vi "vsc_InstallPackage.vi"(8 "error in (no error)":errorcluster, 11 "CommandLine":path) -> (0 "error out":errorcluster, 2 "test details":string, 3 "output to action":string)   [LabVIEW 2017, in "_Try Beta Version of CSMF.lvlib"]
uses:
  _Try Beta Version of CSMF.lvlib
panel:
  out "output to action 2":string
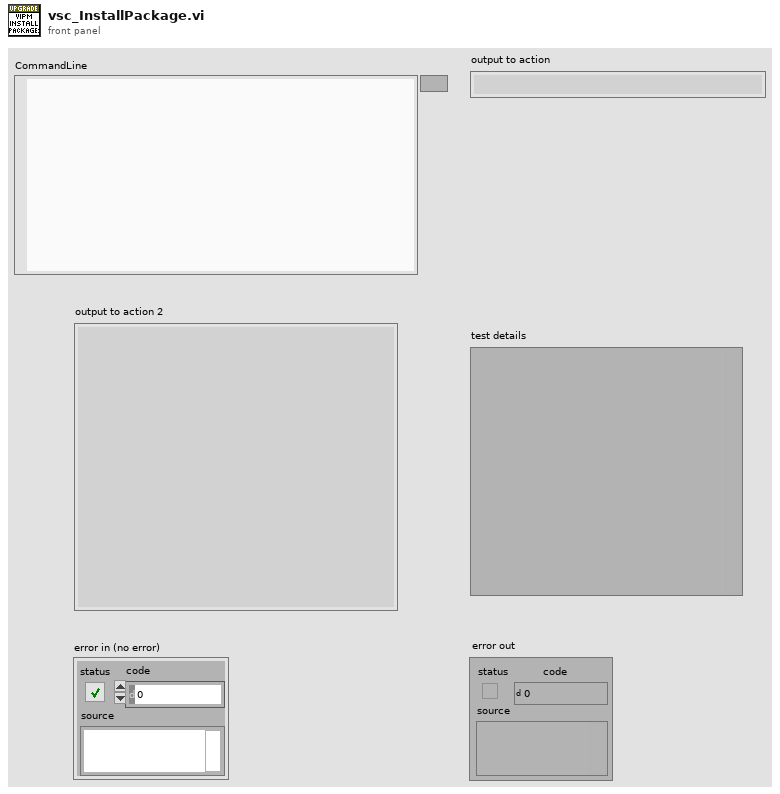
[diagram p1: front panel]
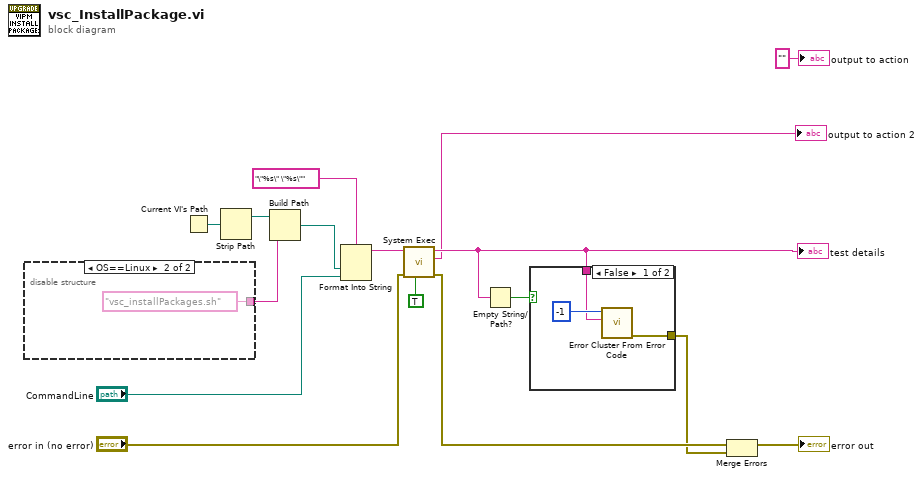
[diagram p0: block diagram]
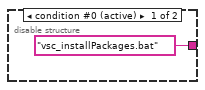
[diagram p2: hidden frame]
diagram:
  n1 = disable-structure shown="OS==Linux" {
    disable-tunnel: ["vsc_installPackages.bat" ("name or relative path") "vsc_installPackages.sh" ("name or relative path")] -> w8
    frame condition #0 (active) {
    }
    frame condition #1 {
    }
  }
  n2 = Current VI's Path() -> (path=w10:path)
  n3 = Strip Path(path=w10) -> (stripped path=w9:path)  [unwired: 1 out]
  n4 = Build Path(base path=w9, name or relative path=w8) -> (appended path=w7:path)
  n5 = Format Into String(format string="\"%s\" \"%s\"" ("command line"), w7, "CommandLine") -> (resulting string=w14:string)  [unwired: 2 in, 1 out]
  n6 = call <vilib>:"System Exec.vi"("run minimized? (F)"=TRUE, "error in (no error)"="error in (no error)", "command line"=w14) -> ("error out"=w11:errorcluster, "standard error"=→"output to action 2":string, "standard output"=w6:string)  [unwired: 5 in, 1 out]
  "test details" <- w6
  n7 = Empty String/Path?(string/path=w6) -> (empty?=w5:bool)
  n8 = case shown="False" w5 {
    tunnel: w6 -> [w20 _]
    tunnel: [w19 _] -> w3
    frame False {
      n9 = call <vilib>:"Error Cluster From Error Code.vi"("error message (\"\")"=w20, "error code (0)"=-1) -> ("error out"=w19:errorcluster)  [unwired: 7 in]
    }
    frame True {
    }
  }
  n10 = Merge Errors(w11, w3) -> (→"error out":errorcluster)
  "output to action" <- "" ("output to action")
